vi "Heal Snake.vi"(8 "error in (no error)":errorcluster, 11 "Snake in":refnum<class "Snake.lvclass">) -> (0 "error out":errorcluster, 3 "Snake out":refnum<class "Snake.lvclass">)   [LabVIEW 2021, in "Snake.lvclass"]
uses:
  Snake.lvclass
  Snake.lvclass/Snake.ctl
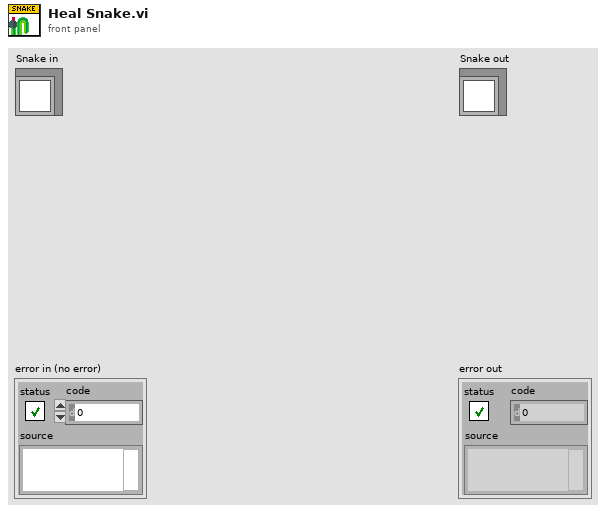
[diagram p1: front panel]
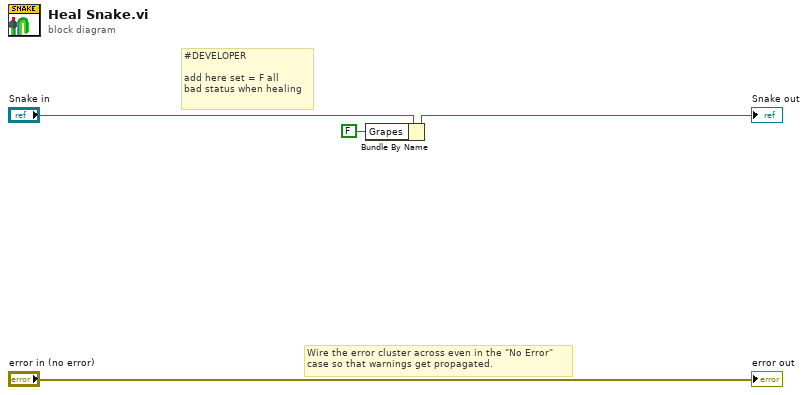
[diagram p0: block diagram]
diagram:
  # "#DEVELOPER\n\nadd here set = F all \nbad status when healing"
  # "Wire the error cluster across even in the \"No Error\"\ncase so that warnings get propagated."
  n1 = Bundle By Name(cluster="Snake in", "Grapes"=FALSE ("Snake Status.Weakeners.Grapes")) -> (→"Snake out":refnum<class "Snake.lvclass">)
  "error out" <- "error in (no error)"
